vi "Get Time from ClockID.vi"(8 "error in (no error)":errorcluster, 11 "CIFCorePlugin in":refnum<class "CIFCorePlugin.lvclass">) -> (0 "error out":errorcluster, 2 "ClockID Time (ns)":u64, 3 "CIFCorePlugin out":refnum<class "CIFCorePlugin.lvclass">)   [LabVIEW 2021, in "CIFCorePlugin.lvclass"]
uses:
  CIFCorePlugin.lvclass
  CIFCorePlugin.lvclass/CIFCorePlugin.ctl
  CIFUtilities/CIFClocks/CIFClocks.lvlib
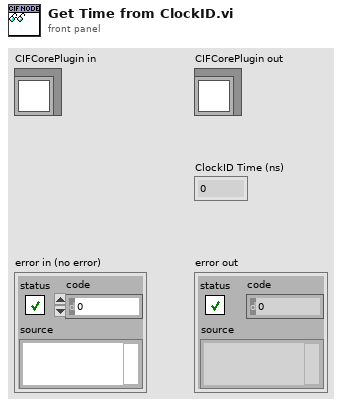
[diagram p1: front panel]
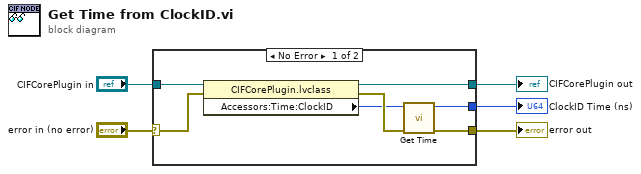
[diagram p0: block diagram]
diagram:
  n1 = case shown="No Error" "error in (no error)" {
    selector: "error in (no error)" -> [w7 w13]
    tunnel: [w6 w13] -> w2
    tunnel: [w8 w14] -> w4
    tunnel: "CIFCorePlugin in" -> [w10 w14]
    tunnel: [w9 _] -> w1
    frame No Error {
      n2 = property class="CIFCorePlugin.lvclass"(reference=w10, error in=w7) -> (reference out=w8:refnum<class "CIFCorePlugin.lvclass">, error out=w12:errorcluster, "Accessors:Time:ClockID"=w11:u8)
      n3 = call "Get Time.vi"("error in (no error)"=w12, "ClockID"=w11) -> ("error out"=w6:errorcluster, "Time (ns)"=w9:u64)  [unwired: 7 in, 1 out]
    }
    frame Error {
    }
  }
  "error out" <- w2
  "CIFCorePlugin out" <- w4
  "ClockID Time (ns)" <- w1
